vi "CHD-simulate-robot-on-field.vi"() -> ()   [LabVIEW 2019]
uses:
  SubVI/CHD_Robot Global Data.vi
  <vilib>/Rock Robotics/WPI/ThirdParty/JAS_Junk/TrajLib/Trajectory_Library.lvlib
  Simulation/CHD_SIM_SIM_Globals.vi
  <vilib>/Rock Robotics/WPI/Camera/WPI_CameraImageSize.ctl
  <vilib>/Rock Robotics/WPI/ThirdParty/JAS_Junk/TrajLib/TypeDef/FieldDisp_ElementPicture.ctl
panel:
  out "ROBOT 2":T1
  in  "Finish":bool
  in  "Enable Vision":bool
  in  "Image Size":T2=enum."320x240"
  out "Field Picture":picture
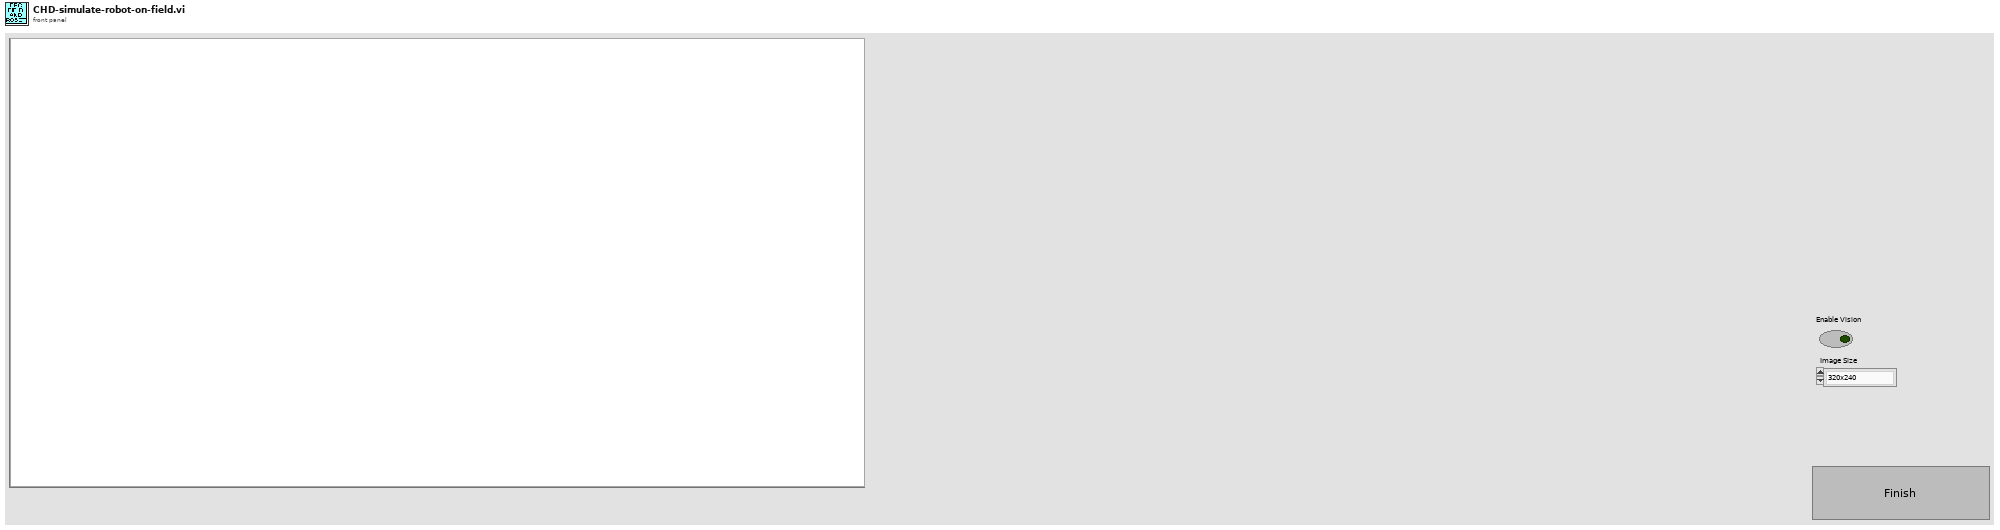
[diagram p1: front panel]
types:
  T1 = typedef "Trajectory_Library.lvlib/FieldDisp_ElementPicture.ctl" = picture
  T2 = typedef "WPI_CameraImageSize.ctl" = enum16{"640x480", "320x240", "160x120", "Custom"}
  T3 = typedef "WPI_DriverStationMatch Info.ctl" = cluster{"Autonomous Elapsed Seconds":dbl, "TeleOp Elapsed Seconds":dbl, "Disabled Elapsed Seconds":dbl, "Visited Autonomous":bool, "Visited TeleOp":bool, "Visited Disabled":bool, "Autonomous Settings":cluster{"Autonomous Style":enum16{"Iterative", "Independent"}, "VI Refnum":refnum<vi>}}
  T4 = typedef "WPI_DriverStationDerivedRobotMode.ctl" = enum16{"Init", "Execute", "Stop"}
  T5 = typedef "WPI_DriverStationRobotMode2.ctl" = enum16{"Autonomous Disabled", "Autonomous Enabled", "Teleop Disabled", "Teleop Enabled", "Disconnected", "Finish", "Test Disabled", "Test Enabled", "Emergency Stopped"}
  T6 = typedef "Trajectory_Library.lvlib/FieldDisp_FieldElement.ctl" = cluster{"ONE-8-bit pixmap":u8[][], "Two-Array":cdb[][], "Three-Numeric":i32, "Four-Numeric":i32, "Five-Numeric":cdb, "Six-colors":u32[], "Seven-new element/subarray":u32, "Left Pixel":dbl, "Top Pixel":dbl, "Width Pix/Ft":dbl, "Height Pix/Ft":dbl, "Element Picture Ref":refnum<vi>}
  T7 = typedef "Trajectory_Library.lvlib/DIFF_DRIVE_ODOM2.ctl" = cluster{"M_POSE_Meters":T8, "M_GyroOffset":T10, "M_PrevAngle":T10, "M_PrevLeftDist_M":dbl, "M_PrevRightDist_M":dbl, "M_InitLeftDist_M":dbl, "M_InitRightDist_M":dbl}
  T8 = typedef "Trajectory_Library.lvlib/POSE2D.ctl" = cluster{"TRANSLATION":T9, "ROTATION":T10}
  T9 = typedef "Trajectory_Library.lvlib/TRANSLATION2D.ctl" = cluster{"X":dbl, "Y":dbl}
  T10 = typedef "Trajectory_Library.lvlib/ROTATION2D.ctl" = cluster{"VALUE":dbl, "COS":dbl, "SIN":dbl}
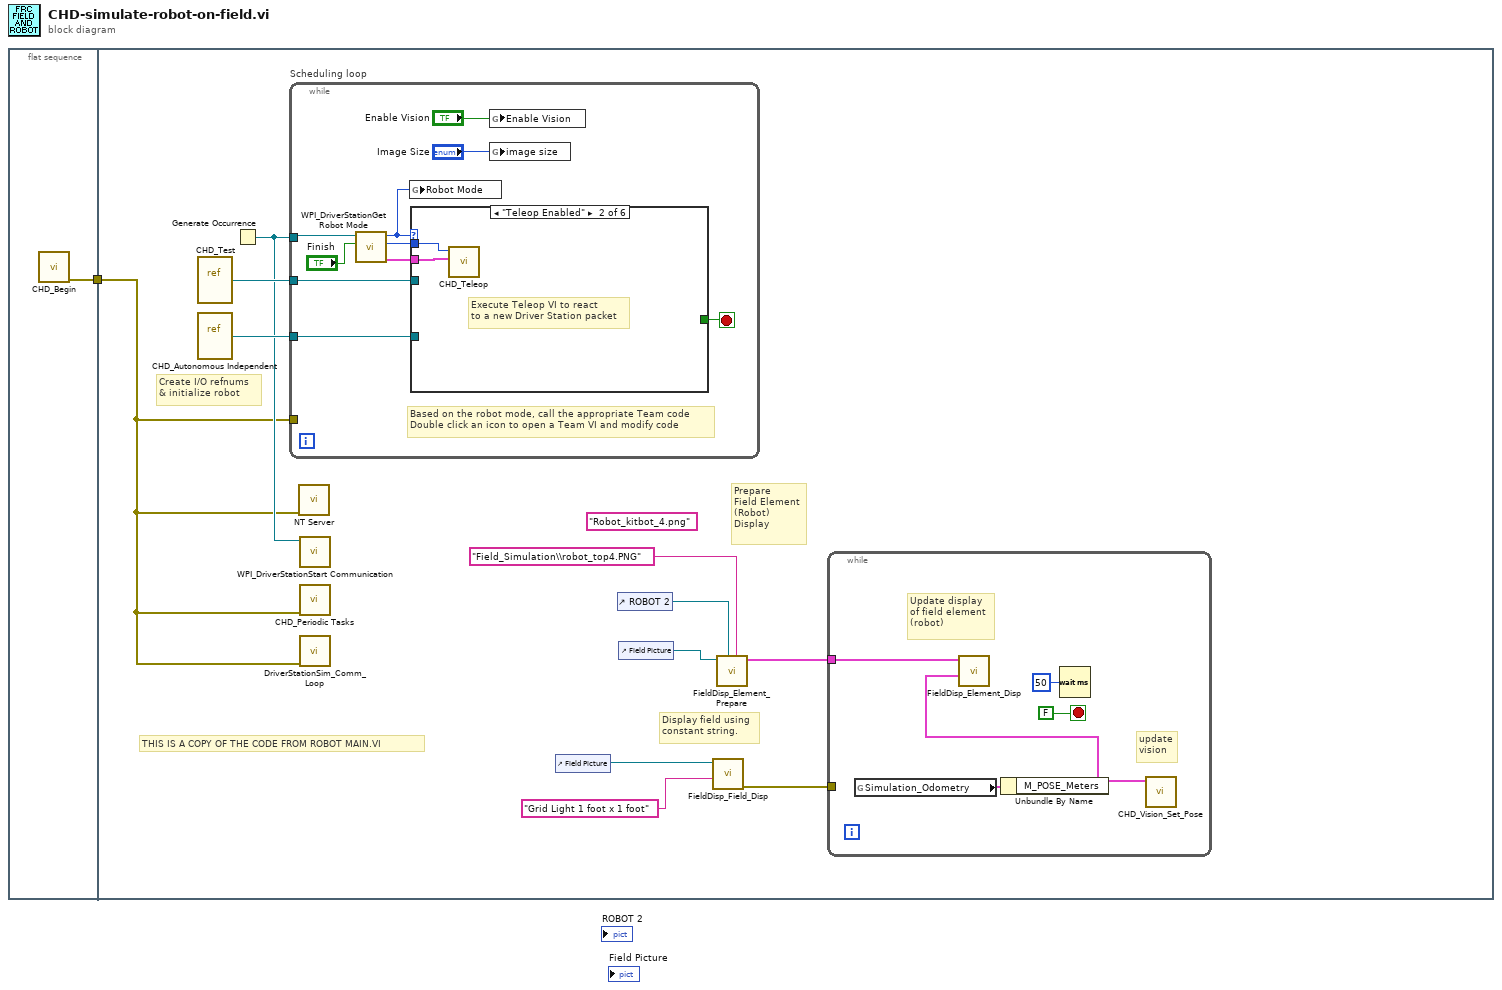
[diagram p0: block diagram]
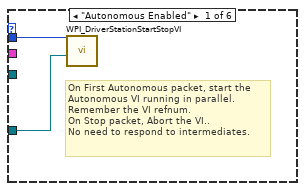
[diagram p2: hidden frame]
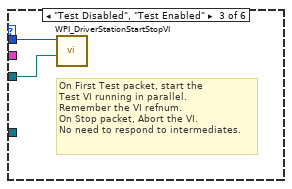
[diagram p3: hidden frame]
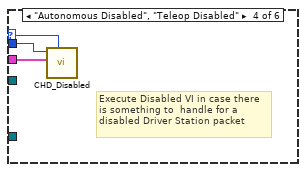
[diagram p4: hidden frame]
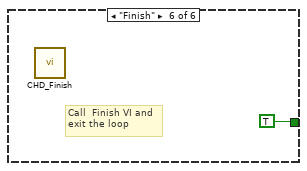
[diagram p6: hidden frame]
diagram:
  n1 = flat-sequence {
    tunnel: [w2] -> w1
    tunnel: w1 -> [w3]
    frame #0 {
      n2 = call "CHD_Begin.vi"() -> ("error out"=w2:errorcluster)  [unwired: 11 in]
    }
    frame #1 {
      (unwired) "Robot_kitbot_4.png" ("Picture FIle Name")
      # "Display field using\nconstant string."
      # "Prepare\nField Element\n(Robot)\nDisplay"
      # "THIS IS A COPY OF THE CODE FROM ROBOT MAIN.VI"
      # "Create I/O refnums\n& initialize robot"
      n3 = vi-ref "CHD_Test.vi"() -> (w12:refnum<vi>)
      n4 = vi-ref "CHD_Autonomous Independent.vi"() -> (w13:refnum<vi>)
      n5 = Generate Occurrence() -> (w11:refnum<k4>)
      n6 = while "Scheduling loop" {
        tunnel: w11 -> [w27]
        tunnel: w3 -> [_]
        tunnel: w13 -> [w22]
        tunnel: w12 -> [w20]
        stop <- w24 stop-if-true
        # "Based on the robot mode, call the appropriate Team code\nDouble click an icon to open a Team VI and modify code"
        n7 = call <vilib>:"WPI_DriverStationGet Robot Mode.vi"("Finish"="Finish", "DS Occurrence"=w27) -> ("Match Info out"=w25:T3, "Call Context"=w28:T4, "Robot Mode"=w19:T5)  [unwired: 7 out]
        n8 = global write "CHD_Robot Global Data.vi" "Robot Mode"(w19) -> ()
        n9 = case shown="\"Teleop Enabled\"" w19 {
          selector: w19 -> [_ _ _ w35 _ _]
          tunnel: w28 -> [w30 w32 w34 w37 _ _]
          tunnel: w25 -> [_ w31 _ w36 _ _]
          tunnel: [_ _ _ _ _ TRUE] -> w24
          tunnel: w22 -> [w29 _ _ _ _ _]
          tunnel: w20 -> [_ _ w33 _ _ _]
          frame "Autonomous Enabled" {
            # "On First Autonomous packet, start the\nAutonomous VI running in parallel.\nRemember the VI refnum.\nOn Stop packet, Abort the VI..\nNo need to respond to intermediates."
            n10 = call <vilib>:"WPI_DriverStationStartStopVI.vi"("VI in"=w29, "Call Context"=w30) -> ()  [unwired: 10 in]
          }
          frame "Teleop Enabled" {
            # "Execute Teleop VI to react\nto a new Driver Station packet"
            n11 = call "CHD_Teleop.vi"("Match Info"=w31, "Call Context"=w32) -> ()  [unwired: 1 in, 9 out]
          }
          frame "Test Disabled", "Test Enabled" {
            # "On First Test packet, start the\nTest VI running in parallel.\nRemember the VI refnum.\nOn Stop packet, Abort the VI.\nNo need to respond to intermediates."
            n12 = call <vilib>:"WPI_DriverStationStartStopVI.vi"("VI in"=w33, "Call Context"=w34) -> ()  [unwired: 10 in]
          }
          frame "Autonomous Disabled", "Teleop Disabled" {
            # "Execute Disabled VI in case there\nis something to  handle for a\ndisabled Driver Station packet"
            n13 = call "CHD_Disabled.vi"("Robot Mode"=w35, "Match Info"=w36, "Call Context"=w37) -> ()  [unwired: 1 in, 8 out]
          }
          frame "Disconnected", Default {
            # "Driver Station packet didn't arrive.\nPossibly useful for diagnostics"
          }
          frame "Finish" {
            # "Call  Finish VI and\nexit the loop"
            n14 = call "CHD_Finish.vi"() -> ()  [unwired: 1 in, 7 out]
          }
        }
        n15 = global write "CHD_Robot Global Data.vi" "Enable Vision"("Enable Vision") -> ()
        n16 = global write "CHD_Robot Global Data.vi" "image size"("Image Size") -> ()
      }
      n17 = call <vilib>:"NT Server.vi"("error in (no error)"=w3) -> ()  [unwired: 10 in, 1 out]
      n18 = call <vilib>:"WPI_DriverStationStart Communication.vi"("occurrence"=w11) -> ()  [unwired: 2 in, 9 out]
      n19 = call "CHD_Periodic Tasks.vi"("error in"=w3) -> ()  [unwired: 11 in]
      n20 = call <vilib>:"DriverStationSim_Comm_Loop.vi"("error in (no error)"=w3) -> ()  [unwired: 11 in]
      n21 = control-ref of="Field Picture"() -> (w7:refnum<vi>)
      n22 = control-ref of="ROBOT 2"() -> (w9:refnum<vi>)
      n23 = control-ref of="Field Picture"() -> (w10:refnum<vi>)
      n24 = call <vilib>:"FieldDisp_Field_Disp.vi"("Field Selector"="Grid Light 1 foot x 1 foot", "Picture in"=w7) -> ("error out"=w6:errorcluster)  [unwired: 9 in]
      n25 = call <vilib>:"FieldDisp_Element_Prepare.vi"("Element File Name"="Field_Simulation\\robot_top4.PNG" ("name or relative path"), "Element Picture Ref"=w9, "Field Picture Ref"=w10) -> ("Field Element Info"=w8:T6)  [unwired: 7 in, 1 out]
      n26 = while {
        tunnel: w8 -> [w16]
        tunnel: w6 -> [_]
        stop <- FALSE stop-if-true
        # "update\nvision"
        # "Update display\nof field element\n(robot)"
        n27 = global read "CHD_SIM_SIM_Globals.vi" "Simulation_Odometry"() -> (w15:T7)
        n28 = Unbundle By Name(w15) -> ("M_POSE_Meters"=w14:T8)
        n29 = call <vilib>:"FieldDisp_Element_Disp.vi"("Element Pose"=w14, "Element Info"=w16) -> ()  [unwired: 10 in]
        n30 = Wait (ms)(milliseconds to wait=u32 50) -> ()  [unwired: 1 out]
        n31 = call "CHD_Vision_Set_Pose.vi"("Vison Pose"=w14) -> ()  [unwired: 11 in]
      }
    }
  }
